vi "X(t).vi"(8 "t":dbl, 11 "A(t)":dbl) -> (3 "X(t)":dbl)   [LabVIEW 2021]
doc: "This VI calculates X(t)"
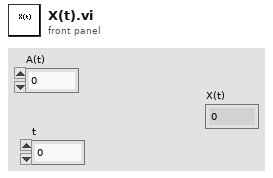
[diagram p1: front panel]
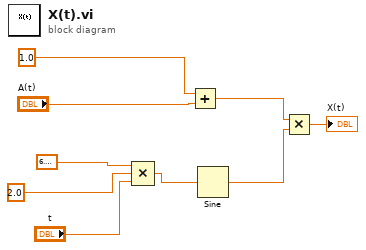
[diagram p0: block diagram]
diagram:
  n1 = Compound Arithmetic op=MULTIPLY(6.283185307179586, 2.0 ("value"), "t") -> (w9:dbl)
  n2 = Add(x=1.0, y="A(t)") -> (x+y=w3:dbl)
  n3 = Sine(x=w9) -> (sin(x)=w2:dbl)
  n4 = Multiply(x=w3, y=w2) -> (x*y=→"X(t)":dbl)
